vi "openbci_test_signals.vi"(10 "Test Signals":T3=45 items=["GND ref"=48, "Slow Sqr 1mV"=45, "Fast Sqr 1mV"=61, "DC signal"=112, "Slow Sqr 2mV"=91, "Fast Sqr 2mV"=93]) -> ()   [LabVIEW 2013]
doc: "Connect all 8 ADS channels to internal test signals.\n 0 inputs shorted to internal ADS1299 ground reference\n - Testing frequency slow, +/-1mV square wave\n = Testing frequency fast, +/-1mV square wave\n p inputs connected to DC signal\n [ Testing frequency slow, +/- 2mV square wave\n [ Testing frequency fast, +/- 2mV square wave"
uses:
  Control Def/test_signals.ctl
  Control Def/openbci_device.ctl
  Control Def/channel_count.ctl
panel:
  in  "error in (no error)":errorcluster
  out "error out":errorcluster
  in  "OBCI dev in":T1={"COM port"="", "n_ch (8)"=enum."8 Channels", "delay_tx"=50}
  out "OBCI dev out":T1={"COM port"="", "n_ch (8)"=enum."8 Channels", "delay_tx"=50}
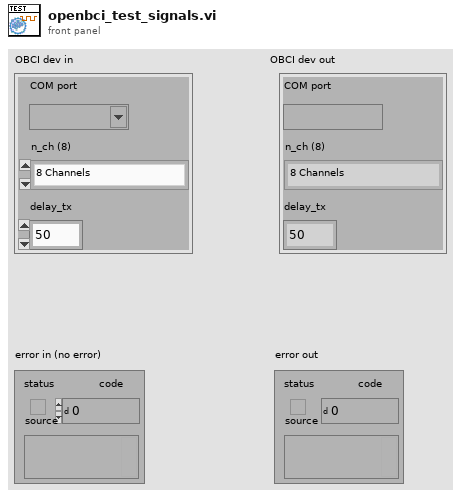
[diagram p1: front panel]
types:
  T1 = typedef "openbci_device.ctl" = cluster{"COM port":refnum<visa-resource-name>, "n_ch (8)":T2, "delay_tx":u32}
  T2 = typedef "channel_count.ctl" = enum16{"8 Channels", "16 Channels"}
  T3 = typedef "test_signals.ctl" = u16
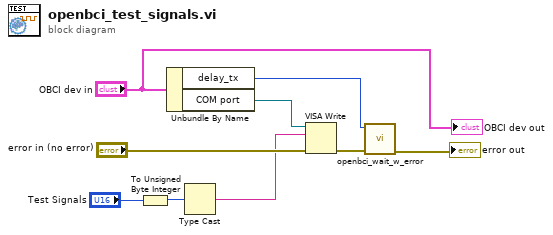
[diagram p0: block diagram]
diagram:
  n1 = To Unsigned Byte Integer(number="Test Signals") -> (unsigned 8bit integer=w8:u8)
  n2 = Unbundle By Name("OBCI dev in") -> ("delay_tx"=w1:u32, "COM port"=w7:refnum<visa-resource-name>)
  n3 = Type Cast(x=w8) -> (*(type *) &x=w4:string)  [unwired: 1 in]
  n4 = VISA Write(VISA resource name=w7, write buffer=w4, error in (no error)="error in (no error)") -> (error out=w3:errorcluster)  [unwired: 2 out]
  n5 = call "openbci_wait_w_error.vi"("error in (no error)"=w3, "milliseconds to wait"=w1) -> ("error out"=→"error out":errorcluster)  [unwired: 9 in]
  "OBCI dev out" <- "OBCI dev in"
